vi "9093_第4回課題_山口修平.vi"() -> ()   [LabVIEW 2020]
panel:
  in  "停止ボタン":bool
  out "波形チャート":dbl(graph)
  out "9000以上":bool
  out "7000以上":bool
  out "出力回数":dbl
  out "乱数(1~10000)":dbl
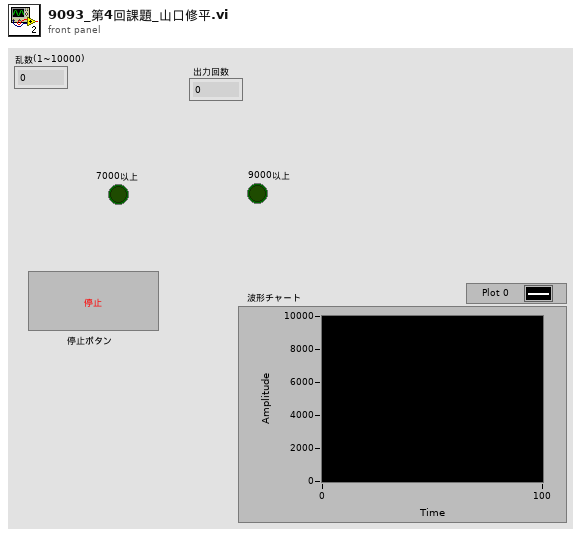
[diagram p1: front panel]
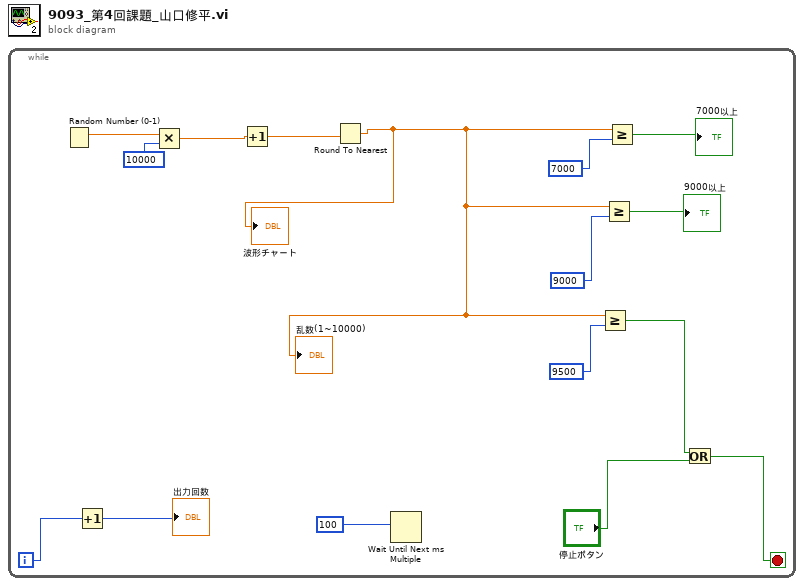
[diagram p0: block diagram]
diagram:
  n1 = while {
    i -> [w8]
    stop <- w10 stop-if-true
    n2 = Random Number (0-1)() -> (number: 0 to 1=w16:dbl)
    n3 = Increment(x=w8) -> (x+1=→"出力回数":i32)
    n4 = Multiply(x=w16, y=10000) -> (x*y=w15:dbl)
    n5 = Increment(x=w15) -> (x+1=w14:dbl)
    n6 = Round To Nearest(number=w14) -> (nearest integer value=w11:dbl)
    "乱数(1~10000)" <- w11
    "波形チャート" <- w11
    n7 = Wait Until Next ms Multiple(millisecond multiple=100) -> ()  [unwired: 1 out]
    n8 = Greater Or Equal?(x=w11, y=9500) -> (x >= y?=w9:bool)
    n9 = Greater Or Equal?(x=w11, y=9000) -> (x >= y?=→"9000以上":bool)
    n10 = Greater Or Equal?(x=w11, y=7000) -> (x >= y?=→"7000以上":bool)
    n11 = Or(x=w9, y="停止ボタン") -> (x .or. y?=w10:bool)
  }
